vi "Initialize piezo driver.vi"(8 "error in (no error)":errorcluster, 10 "Set piezo to 0V":dbl, 11 "COM port in":refnum<visa-resource-name>) -> (0 "error out":errorcluster, 2 "Voltage range":i32, 3 "COM port out":refnum<visa-resource-name>)   [LabVIEW 2020]
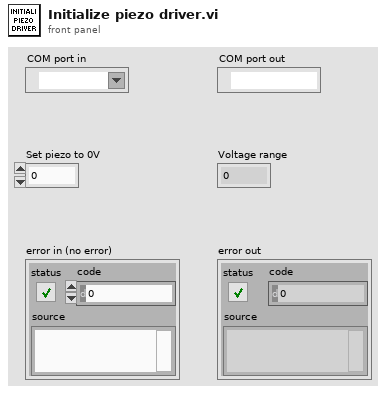
[diagram p1: front panel]
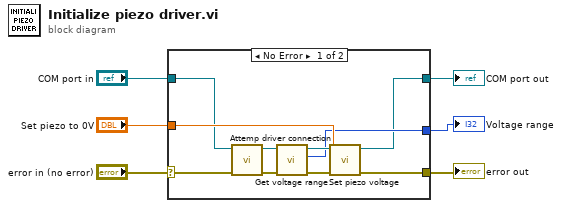
[diagram p0: block diagram]
diagram:
  n1 = case shown="No Error" "error in (no error)" {
    selector: "error in (no error)" -> [w8 w17]
    tunnel: "Set piezo to 0V" -> [w16 _]
    tunnel: [w14 w17] -> w5
    tunnel: [w12 _] -> w4
    tunnel: "COM port in" -> [w9 w18]
    tunnel: [w7 w18] -> w1
    frame No Error {
      n2 = call "Attemp driver connection.vi"("error in (no error)"=w8, "COM port in"=w9) -> ("error out"=w10:errorcluster, "COM port out"=w11:refnum<visa-resource-name>)  [unwired: 8 in]
      n3 = call "Get voltage range.vi"("error in (no error)"=w10, "COM port in"=w11) -> ("error out"=w13:errorcluster, "Voltage range"=w12:i32, "COM port out"=w15:refnum<visa-resource-name>)  [unwired: 7 in]
      n4 = call "Set piezo voltage.vi"("error in (no error)"=w13, "Voltage"=w16, "COM port in"=w15) -> ("error out"=w14:errorcluster, "COM port out"=w7:refnum<visa-resource-name>)  [unwired: 7 in]
    }
    frame Error {
    }
  }
  "error out" <- w5
  "Voltage range" <- w4
  "COM port out" <- w1
